vi "Initialize Actor.vi"(7 "Host Name":string, 8 "error in (no error)":errorcluster, 9 "Actor Name":string, 10 "Message Broker Interface":refnum<class "Message Broker Interface.lvclass">, 11 "Terminal Menus in":refnum<class "Terminal Menus.lvclass">) -> (0 "error out":errorcluster, 3 "Terminal Menus out":refnum<class "Terminal Menus.lvclass">)   [LabVIEW 2016, in "CLD Exam - ATM.lvlib" / "Terminal Menus.lvclass"]
uses:
  Terminal Menus.lvclass
  Mediator/Classes/Message Broker Interface/Message Broker Interface.lvclass
  Terminal Menus.lvclass/Terminal Menus.ctl
  Mediator/Classes/Message Transport Event/Message Transport Event.lvclass
  D:/Repos/Stream/software/Mediator/Classes/Message Transport Interface/Message Transport Interface.lvclass
  Mediator/Classes/Mediated Synchronous Actor/Mediated Synchronous Actor.lvclass
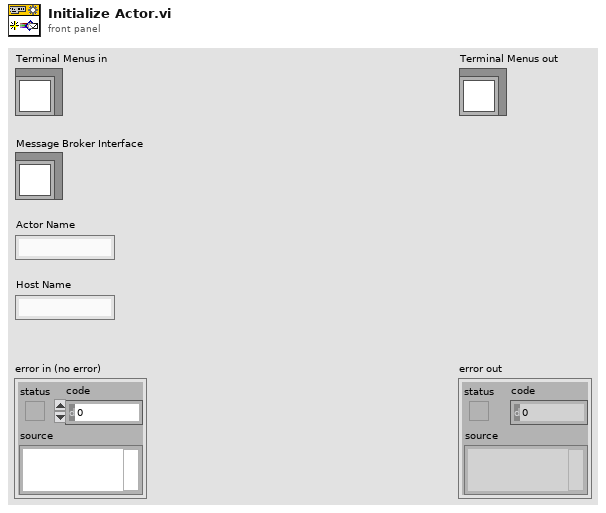
[diagram p1: front panel]
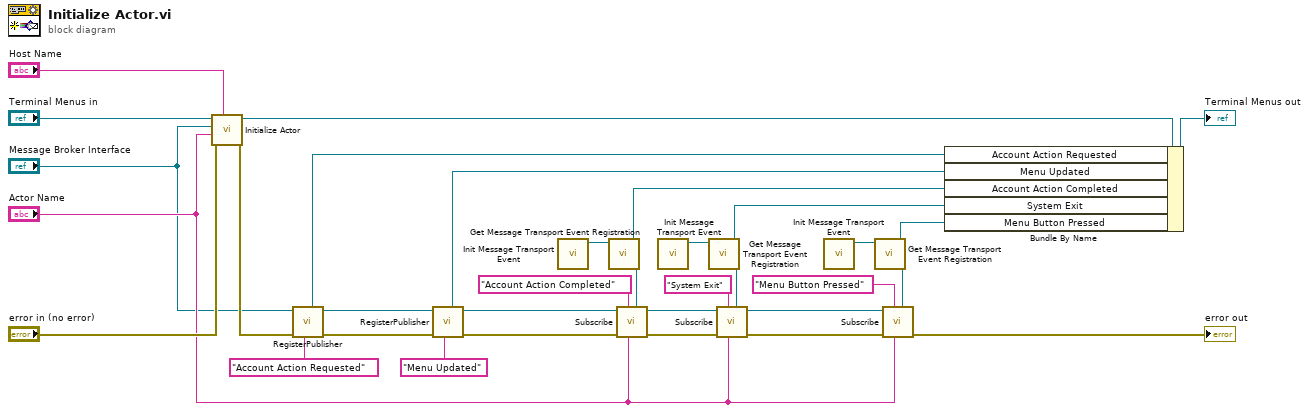
[diagram p0: block diagram]
diagram:
  n1 = call-parent "Initialize Actor.vi"("Host Name"="Host Name", "error in (no error)"="error in (no error)", "Actor Name"="Actor Name", "Message Broker Interface"="Message Broker Interface", "Mediated Synchronous Actor in"="Terminal Menus in") -> ("error out"=w5:errorcluster, "Mediated Synchronous Actor out"=w29:refnum<class "Terminal Menus.lvclass">)  [unwired: 5 in]
  n2 = call-dynamic "RegisterPublisher.vi"("Topic Name"="Account Action Requested", "error in (no error)"=w5, "Message Broker Interface in"="Message Broker Interface") -> ("error out"=w4:errorcluster, "Message Broker Interface out"=w2:refnum<class "Message Broker Interface.lvclass">, "Transport"=w1:refnum<class "Message Transport Queue.lvclass">)  [unwired: 4 in, 2 out]
  n3 = call-dynamic "RegisterPublisher.vi"("Topic Name"="Menu Updated", "error in (no error)"=w4, "Message Broker Interface in"=w2) -> ("error out"=w21:errorcluster, "Message Broker Interface out"=w22:refnum<class "Message Broker Interface.lvclass">, "Transport"=w26:refnum<class "Message Transport Queue.lvclass">)  [unwired: 4 in, 2 out]
  n4 = call "Init Message Transport Event.vi"() -> ("Message Transport Event out"=w23:refnum<class "Message Transport Event.lvclass">)  [unwired: 10 in, 1 out]
  n5 = call "Get Message Transport Event Registration.vi"("Message Transport Event in"=w23) -> ("Event Registration Refnum"=w20:refnum<event-registration>, "Message Transport Event out"=w24:refnum<class "Message Transport Event.lvclass">)  [unwired: 7 in, 2 out]
  n6 = call-dynamic "Subscribe.vi"("Message Transport Interface"=w24, "Subscriber Name"="Actor Name", "Topic Name"="Account Action Completed", "error in (no error)"=w21, "Message Broker Interface in"=w22) -> ("error out"=w15:errorcluster, "Message Broker Interface out"=w16:refnum<class "Message Broker Interface.lvclass">)  [unwired: 4 in, 1 out]
  n7 = call "Init Message Transport Event.vi"() -> ("Message Transport Event out"=w19:refnum<class "Message Transport Event.lvclass">)  [unwired: 10 in, 1 out]
  n8 = call "Get Message Transport Event Registration.vi"("Message Transport Event in"=w19) -> ("Event Registration Refnum"=w14:refnum<event-registration>, "Message Transport Event out"=w18:refnum<class "Message Transport Event.lvclass">)  [unwired: 7 in, 2 out]
  n9 = call-dynamic "Subscribe.vi"("Message Transport Interface"=w18, "Subscriber Name"="Actor Name", "Topic Name"="System Exit", "error in (no error)"=w15, "Message Broker Interface in"=w16) -> ("error out"=w9:errorcluster, "Message Broker Interface out"=w10:refnum<class "Message Broker Interface.lvclass">)  [unwired: 4 in, 1 out]
  "error out" <- w9
  n10 = call "Init Message Transport Event.vi"() -> ("Message Transport Event out"=w11:refnum<class "Message Transport Event.lvclass">)  [unwired: 10 in, 1 out]
  n11 = call "Get Message Transport Event Registration.vi"("Message Transport Event in"=w11) -> ("Event Registration Refnum"=w7:refnum<event-registration>, "Message Transport Event out"=w12:refnum<class "Message Transport Event.lvclass">)  [unwired: 7 in, 2 out]
  n12 = call-dynamic "Subscribe.vi"("Message Transport Interface"=w12, "Subscriber Name"="Actor Name", "Topic Name"="Menu Button Pressed", "error in (no error)"=w9, "Message Broker Interface in"=w10) -> ()  [unwired: 4 in, 3 out]
  n13 = Bundle By Name(cluster=w29, "Account Action Requested"=w1, "Menu Updated"=w26, "Account Action Completed"=w20, "System Exit"=w14, "Menu Button Pressed"=w7) -> (→"Terminal Menus out":refnum<class "Terminal Menus.lvclass">)
